vi "adjustdataacqsize.vi"(3 "waveform size in":i32) -> (0 "waveform size out":dbl, 1 "# of points":i32)   [LabVIEW 2015]
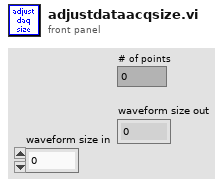
[diagram p1: front panel]
types:
  T1 = typedef "LVRectTypeDef.ctl" = cluster{"Left":i16, "Top":i16, "Right":i16, "Bottom":i16}
  T2 = cluster{"Xpixels":i32, "Vxminref":dbl, "Vxmaxref":dbl, "P":dbl, "Ypixels":i32, "Vyminref":dbl, "Vymaxref":dbl, "srate":sgl, "sAOxy":i32, "timeout":dbl, "type":string, "date":string, "time":string, "Colormap":u16, "Drawing Mode":u16, "Scanning Mode":u16, "square pixels":bool, "square matrix":bool, "Xpixels Img":i32, "Vx-min Img":dbl, "VX-max Img":dbl, "Ypixels Img":i32, "Vy-min Img":dbl, "Vy-max Img ":dbl, "Angle Img":dbl, "autoshutter":bool, "finite":bool, "cont":bool, "wavdet":bool, "measpoints":i32, "avpp":i32, "bufferAO":i32, "bufferAI":i32, "starttick":u32, "waveform":path, "Vx-ref":dbl, "Vy-ref":dbl, "refreshrate":dbl, "refreshbuffer":i32, "tt_cycles":i32, "motorref":refnum<k7>, "mirrorswitch":refnum<k7>, "sample mode":i32, "maxbufferAI":i32, "srateAODO":sgl, "bin":sgl, "Pel":sgl, "Angle draw":dbl, "srate Img":sgl, "ROIimg_plotbounds":T1, "auto OD":bool, "ODfilt":u16, "aAI":i32[], "aCI":i32[], "aAO":u32[], "aDO":u32[], "refwfsize":dbl, "Lifetime":bool, "Vz-Img":dbl, "Vz-ref":dbl, "Vz-reset":dbl, "AIoverride":bool}
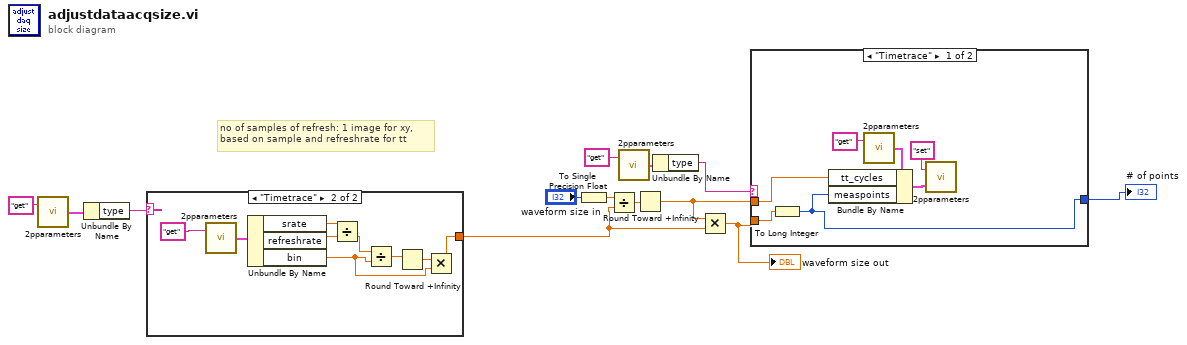
[diagram p0: block diagram]
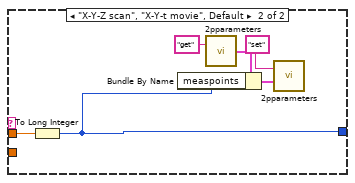
[diagram p2: hidden frame]
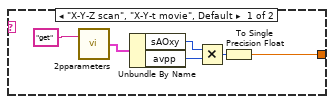
[diagram p3: hidden frame]
diagram:
  # "no of samples of refresh: 1 image for xy, \nbased on sample and refreshrate for tt"
  n1 = call "2pparameters.vi"("command"="get") -> ("params out"=w7:T2)  [unwired: 1 in]
  n2 = Unbundle By Name(w7) -> ("type"=w8:string)
  n3 = case shown="\"Timetrace\"" w8 {
    tunnel: [w14 w20] -> w9
    frame "X-Y-Z scan", "X-Y-t movie", Default {
      n4 = call "2pparameters.vi"("command"="get") -> ("params out"=w18:T2)  [unwired: 1 in]
      n5 = Unbundle By Name(w18) -> ("sAOxy"=w17:i32, "avpp"=w16:i32)
      n6 = Multiply(x=w17, y=w16) -> (x*y=w15:i32)
      n7 = To Single Precision Float(number=w15) -> (single precision float=w14:sgl)
    }
    frame "Timetrace" {
      n8 = call "2pparameters.vi"("command"="get") -> ("params out"=w26:T2)  [unwired: 1 in]
      n9 = Unbundle By Name(w26) -> ("srate"=w28:sgl, "refreshrate"=w27:dbl, "bin"=w21:sgl)
      n10 = Divide(x=w28, y=w27) -> (x/y=w24:dbl)
      n11 = Divide(x=w24, y=w21) -> (x/y=w23:dbl)
      n12 = Round Toward +Infinity(x=w23) -> (ceil(x): smallest int >= x=w22:dbl)
      n13 = Multiply(x=w22, y=w21) -> (x*y=w20:dbl)
    }
  }
  n14 = To Single Precision Float(number="waveform size in") -> (single precision float=w4:sgl)
  n15 = Divide(x=w4, y=w9) -> (x/y=w3:dbl)
  n16 = call "2pparameters.vi"("command"="get") -> ("params out"=w11:T2)  [unwired: 1 in]
  n17 = Round Toward +Infinity(x=w3) -> (ceil(x): smallest int >= x=w2:dbl)
  n18 = Unbundle By Name(w11) -> ("type"=w13:string)
  n19 = Multiply(x=w2, y=w9) -> (x*y=w10:dbl)
  "waveform size out" <- w10
  n20 = case shown="\"Timetrace\"" w13 {
    tunnel: w2 -> [w30 w37]
    tunnel: w10 -> [w35 _]
    tunnel: [w29 w36] -> w1
    frame "Timetrace" {
      n21 = To Long Integer(number=w35) -> (32bit integer=w29:i32)
      n22 = call "2pparameters.vi"("command"="get") -> ("params out"=w33:T2)  [unwired: 1 in]
      n23 = Bundle By Name(cluster=w33, "tt_cycles"=w30, "measpoints"=w29) -> (w31:T2)
      n24 = call "2pparameters.vi"("Params in"=w31, "command"="set") -> ()  [unwired: 1 out]
    }
    frame "X-Y-Z scan", "X-Y-t movie", Default {
      n25 = To Long Integer(number=w37) -> (32bit integer=w36:i32)
      n26 = call "2pparameters.vi"("command"="get") -> ("params out"=w41:T2)  [unwired: 1 in]
      n27 = Bundle By Name(cluster=w41, "measpoints"=w36) -> (w39:T2)
      n28 = call "2pparameters.vi"("Params in"=w39, "command"="set") -> ()  [unwired: 1 out]
    }
  }
  "# of points" <- w1
